vi "PQfinish.vi"(8 "error in (no error)":errorcluster, 10 "conn":u32) -> (0 "error out":errorcluster)   [LabVIEW 2018, in "libpqlv.lvlib"]
doc: "Closes the connection to the server. Also frees memory used by the PGconn object."
uses:
  libpqlv.lvlib
  lib/libpq.dll
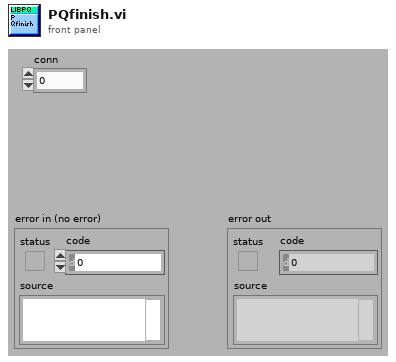
[diagram p1: front panel]
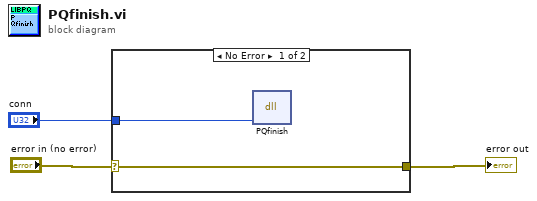
[diagram p0: block diagram]
diagram:
  n1 = case shown="No Error" "error in (no error)" {
    selector: "error in (no error)" -> [w5 w6]
    tunnel: [w5 w6] -> w2
    tunnel: "conn" -> [w4 _]
    frame No Error {
      n2 = dll-call lib="D:/Users/erics/Documents/TC-3/DAQ/PostgreSQL2LabVIEW/libpqlv/lib/libpq.*" fn="PQfinish"("conn"=w4) -> ()  [unwired: 5 in, 2 out]
    }
    frame Error {
    }
  }
  "error out" <- w2
